vi "Main.vi"() -> ()   [LabVIEW 2015]
uses:
  Math Library/Math Library.lvlib
panel:
  out "X+Y":dbl
  in  "y":dbl
  # "Nancy Change"
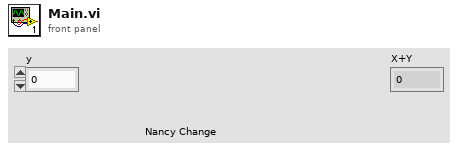
[diagram p1: front panel]
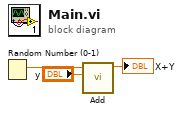
[diagram p0: block diagram]
diagram:
  n1 = Random Number (0-1)() -> (number: 0 to 1=w3:dbl)
  n2 = call "Add.vi"("y"="y", "x"=w3) -> ("X+Y"=→"X+Y":dbl)  [unwired: 9 in]
